vi "tomaDatos.vi"() -> ()   [LabVIEW 2017]
panel:
  in  "stop":bool
  out "Temperatura 2":dbl
  out "Voltaje Salida Amplificador 2":dbl
  out "Temperatura 1":dbl
  out "Voltaje Salida Amplificador 1":dbl
  out "Temperatura 2":dynamicdata(graph)
  out "Temperatura 1":dynamicdata(graph)
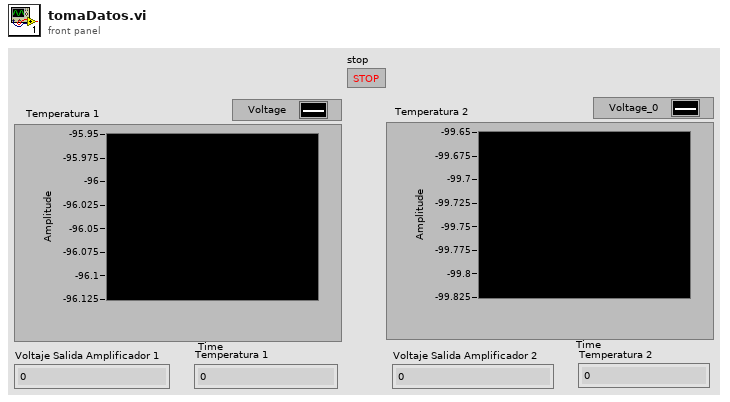
[diagram p1: front panel]
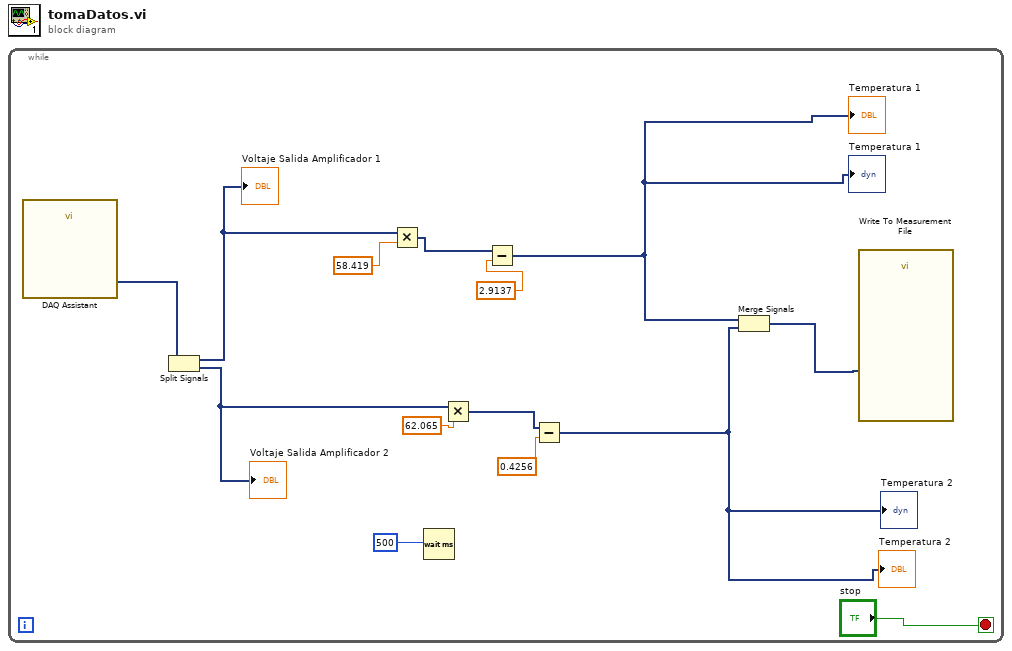
[diagram p0: block diagram]
diagram:
  n1 = while {
    stop <- "stop" stop-if-true
    n2 = call "DAQ Assistant"() -> ("data"=w1:dynamicdata)  [unwired: 17 in, 2 out]
    n3 = Split Signals(w1) -> (w9:dynamicdata, w8:dynamicdata)  [unwired: 2 in]
    "Voltaje Salida Amplificador 1" <- w9
    "Voltaje Salida Amplificador 2" <- w8
    n4 = Multiply(x=w9, y=58.419) -> (x*y=w7:dynamicdata)
    n5 = Wait (ms)(milliseconds to wait=500) -> ()  [unwired: 1 out]
    n6 = Multiply(x=w8, y=62.065) -> (x*y=w4:dynamicdata)
    n7 = Subtract(x=w7, y=2.9137) -> (x-y=w5:dynamicdata)
    "Temperatura 1" <- w5
    "Temperatura 1" <- w5
    n8 = Subtract(x=w4, y=0.4256) -> (x-y=w3:dynamicdata)
    "Temperatura 2" <- w3
    "Temperatura 2" <- w3
    n9 = Merge Signals(w5, w3) -> (w14:dynamicdata)
    n10 = call "Write To Measurement File"("Signals"=w14) -> ()  [unwired: 16 in, 3 out]
  }
